vi "TEST - Get Strings from Enum TD.vi"(8 "error in (no error)":errorcluster) -> (0 "error out":errorcluster, 2 "pass":bool)   [LabVIEW 2020]
uses:
  source/library/openg_variant.lvlib
panel:
  out "Failures":T1(array[cluster])
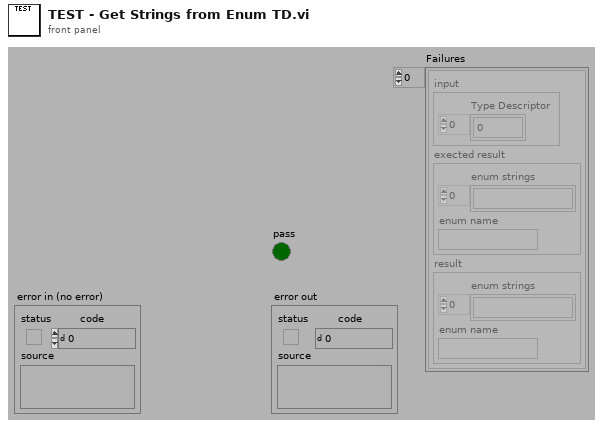
[diagram p1: front panel]
types:
  T1 = cluster{"input":cluster{"Type Descriptor":i16[]}, "exected result":cluster{"enum strings":string[], "enum name":string}, "result":cluster{"enum strings":string[], "enum name":string}}[]
  T2 = cluster{"input":cluster{"Type Descriptor":i16[]}, "exected result":cluster{"enum strings":string[], "enum name":string}, "result":cluster{"enum strings":string[], "enum name":string}}
  T3 = cluster{"enum strings":string[], "enum name":string}
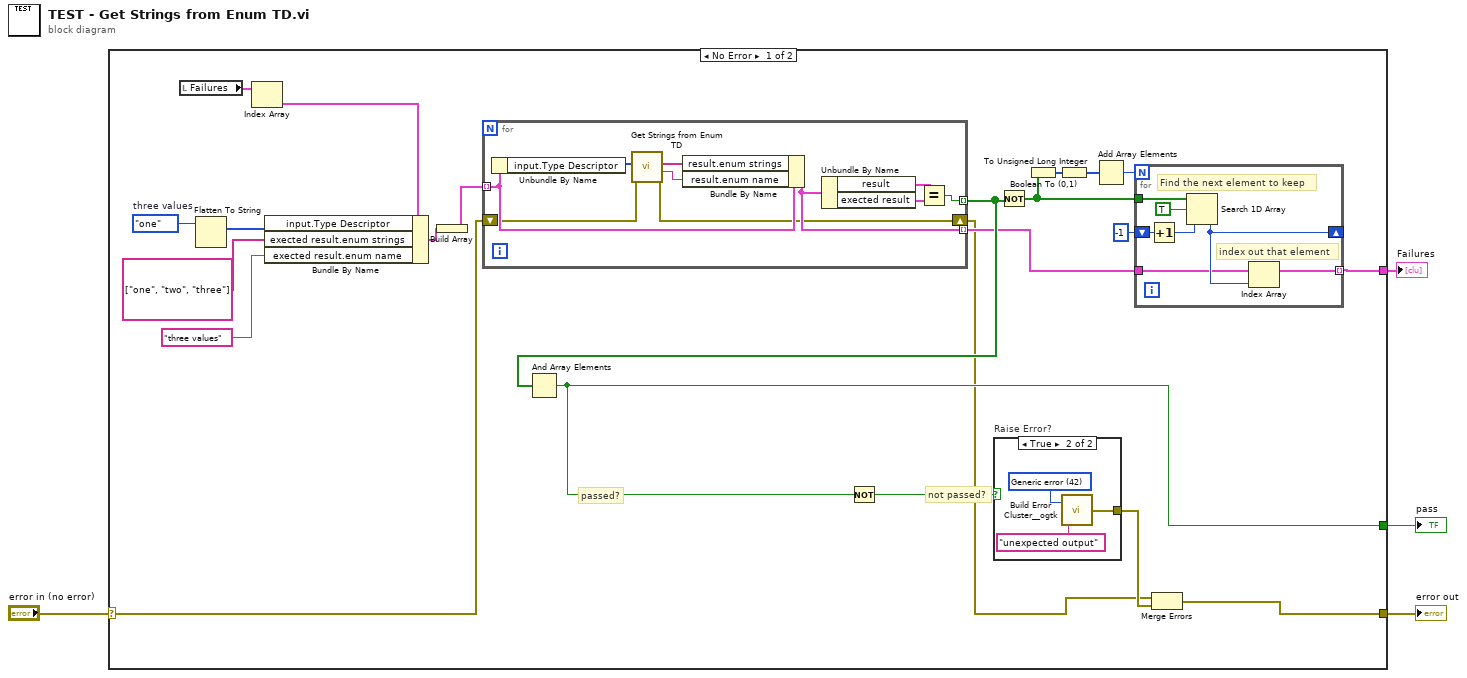
[diagram p0: block diagram]
diagram:
  n1 = case shown="No Error" "error in (no error)" {
    selector: "error in (no error)" -> [w12 w47]
    tunnel: [w23 _] -> w4
    tunnel: [w26 w47] -> w2
    tunnel: [w15 _] -> w1
    frame No Error {
      w8 = enum16{"one", "two", "three"}."one"  # three values
      # "not passed?"
      # "passed?"
      n2 = local read "Failures"() -> (w10:T1)
      n3 = Flatten To String(anything=w8) -> (type string=w7:i16[])  [unwired: 3 in, 2 out]
      n4 = Index Array(array=w10) -> (element=w9:T2)  [unwired: 1 in]
      n5 = Bundle By Name(cluster=w9, "input.Type Descriptor"=w7, "exected result.enum strings"=string[] ["one", "two", "three"], "exected result.enum name"="three values") -> (w14:T2)
      n6 = Build Array(w14) -> (w13:T1)
      n7 = for {
        tunnel: w13 -> [w42] mode=indexing
        tunnel: [w43] -> w17 mode=indexing
        tunnel: [w41] -> w16 mode=indexing
        shift-right: [w38] -> w11
        shift-left: w12 -> [w37]
        n8 = Unbundle By Name(w42) -> ("input.Type Descriptor"=w36:i16[])
        n9 = call "Get Strings from Enum TD.vi"("error in (no error)"=w37, "Type Descriptor"=w36) -> ("error out"=w38:errorcluster, "enum name"=w34:string, "enum strings"=w35:string[])  [unwired: 7 in]
        n10 = Bundle By Name(cluster=w42, "result.enum strings"=w35, "result.enum name"=w34) -> (w41:T2)
        n11 = Unbundle By Name(w41) -> ("result"=w40:T3, "exected result"=w39:T3)
        n12 = Equal?(x=w40, y=w39) -> (x = y?=w43:bool)
      }
      n13 = And Array Elements(Boolean array=w17) -> (logical AND=w23:bool)
      n14 = Not(x=w23) -> (.not. x?=w24:bool)
      n15 = case "Raise Error?" shown="True" w24 {
        tunnel: [_ w44] -> w25
        frame False {
        }
        frame True {
          w45 = 42 items=["No error", "Argument error", "Memory is full", "Out of zone", "End of file", "File already open", "Generic file I/O error", "File not found", "File permission error", "Disk is full", "Duplicate path", "Too many files open", "System feature not enabled", "Resource file not found", "Cannot add resource", "Resource not found", "Image not found", "Image memory error", "Pen does not exist", "Config type invalid", "Config token not found", "Config parse error", "Config memory error", "Bad external code format", "Bad external code offset", "External code not present", "Null window", "Destroy window error", "Null menu", "Print aborted", "Bad print record", "Print driver error", "Windows error during printing", "Memory error during printing", "Print dialog error", "Generic print error", "Invalid device refnum", "Device not found", "Device parameter error", "Device unit error", "Cannot open device", "Device call aborted", "Generic error", "Cancelled by user", "Object ID too low", "Object ID too high", "Object not in heap", "Unknown heap", "Unknown object (invalid DefProc)", "Unknown object (DefProc not in table)", "Message out of range", "Invalid (null) method", "Unknown message", "Manager call not supported", "Bad address", "Network operation in progress", "Network operation timed out", "Connection is busy", "Network attribute not supported", "Network error", "Address in use", "System out of memory", "Connection aborted", "Connection refused", "Not connected", "Already connected", "Connection closed", "Initialization error (interapplication manager)", "Bad occurrence", "Wait on unbound occurrence handler", "Occurrence queue overflow", "Datalog type conflict", "Unused", "Unrecognized type (interapplication manager)", "Memory corrupt", "Failed to make temporary DLL", "Old CIN version", "Drag socket not found", "Failed to load drop-object", "Failed to register OLE object", "Failed to release OLE object", "Format specifier type mismatch", "Unknown format specifier", "Too few format specifiers", "Too many format specifiers", "Scan failed", "Newer CIN version", "Error converting to variant", "Runtime menu error", "Password tampered", "Variant attribute not found", "Incompatible variant data type", "Event data is not available", "Event Store is not present", "Occurrence is not found", "Event Queue is not created", "Event info is not available", "Refnum passed is NULL", "Error retrieving Class GUID", "Error retrieving CoClass GUID", "Error retrieving TypeLib GUID.", "Bad built application magic bytes.", "Specific driver is different from the specific driver associated with the Logical Name.", "There is no session opened to the class driver.", "Max Error", "MAX - Error with config objects", "MAX - Error loading configuration", "MAX - Group not supported"]
          n16 = call <userlib>:"Build Error Cluster__ogtk.vi"("String to Prepend to source (\"\")"="unexpected output" ("String to Prepend to source (\"\")"), "code"=w45) -> ("error out"=w44:errorcluster)
        }
      }
      n17 = Not(x=w17) -> (.not. x?=w19:bool[])
      n18 = Boolean To (0,1)(Boolean=w19) -> (0, 1=w20:i16[])
      n19 = To Unsigned Long Integer(number=w20) -> (unsigned 32bit integer=w18:u32[])
      n20 = Add Array Elements(numeric array=w18) -> (sum=w21:u32)
      n21 = for {
        N: w21 -> [_]
        tunnel: w16 -> [w29]
        tunnel: w19 -> [w33]
        shift-right: [w30] -> _
        shift-left: -1 ("start index (0)") -> [w31]
        tunnel: [w28] -> w15 mode=indexing
        # "index out that element"
        # "Find the next element to keep"
        n22 = Increment(x=w31) -> (x+1=w27:i32)
        n23 = Search 1D Array(1D array=w33, element=TRUE, start index (0)=w27) -> (index of element=w30:i32)
        n24 = Index Array(array=w29, index=w30) -> (element=w28:T2)
      }
      n25 = Merge Errors(w11, w25) -> (w26:errorcluster)
    }
    frame Error {
    }
  }
  "pass" <- w4
  "error out" <- w2
  "Failures" <- w1
